vi "Load Calibration Image.vi"(10 "File Path":path=path "C:/ProgramData/Vision/Config/cam6/cam6 calibration.png", 11 "Camera Name":string="Image Calibration 1") -> (0 "error out":errorcluster, 1 "Internal Parameters":T3, 2 "Calibration Axis Info":T2, 3 "Image Out":T1, 4 "Distortion Model Coefficients":T4={"Distortion Model"=-1, "Polynomial Coefficients"={"Radial Coefficients"=[], "Tangential Coefficients"={"P1"=0.0, "P2"=0.0}}, "Division Model kappa"=0.0} {"Distortion Model" items=["None"=-1, "Polynomial"=0, "Division"=1]})   [LabVIEW 2025]
uses:
  <vilib>/vision/Image Controls.llb/IMAQ Image.ctl
  <vilib>/vision/Calibration.llb/Distortion Model Coefficients.ctl
  <vilib>/vision/Calibration.llb/Distortion Model Types.ctl
  <vilib>/vision/Calibration.llb/Internal Parameters.ctl
  <vilib>/vision/NI_Vision_Development_Module.lvlib
panel:
  out "Calibration Camera Image":T1(plugin-control)
  in  "error in":errorcluster
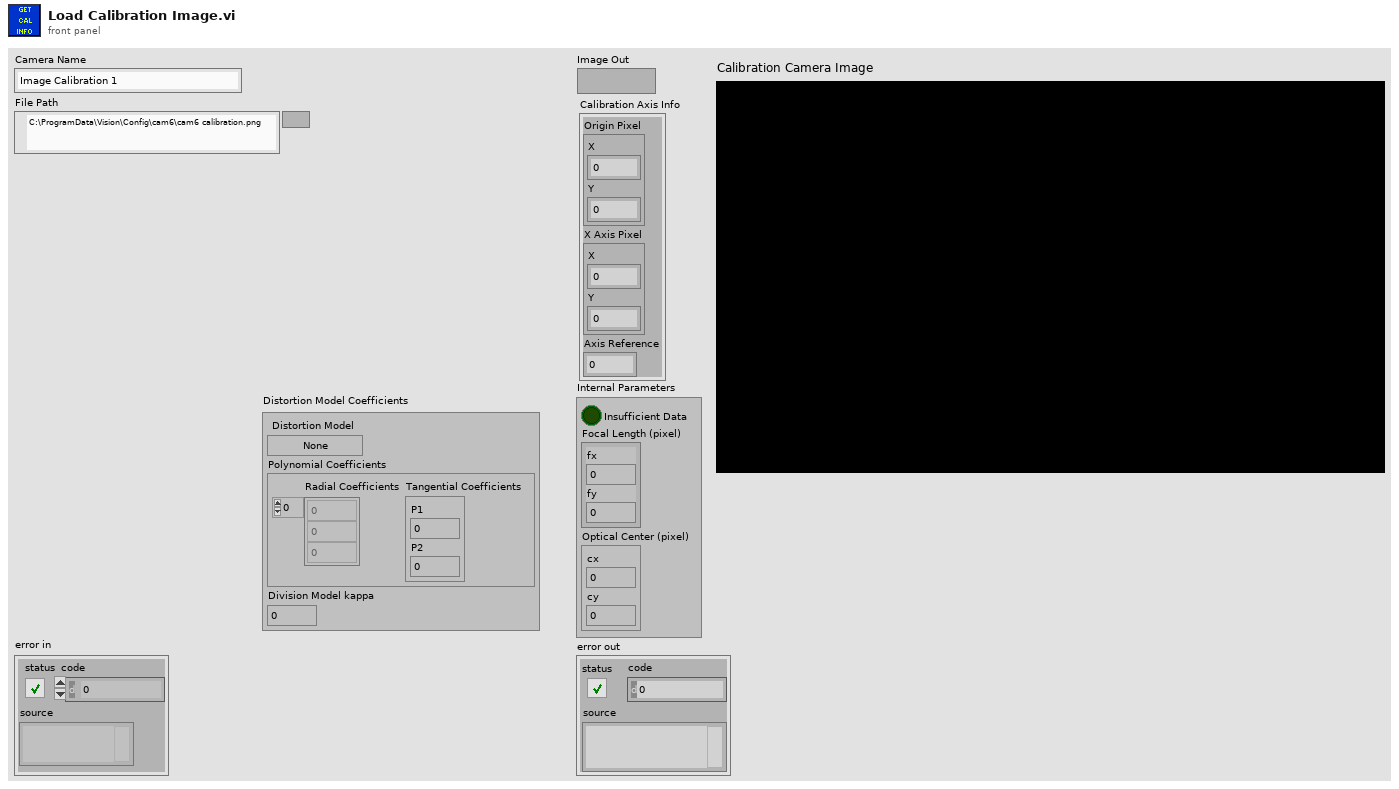
[diagram p1: front panel]
types:
  T1 = typedef "IMAQ Image.ctl" = refnum<image>
  T2 = cluster{"Origin Pixel":cluster{"X":sgl, "Y":sgl}, "X Axis Pixel":cluster{"X":sgl, "Y":sgl}, "Axis Reference":u32}
  T3 = typedef "Internal Parameters.ctl" = cluster{"Insufficient Data":bool, "Focal Length (pixel)":cluster{"fx":sgl, "fy":sgl}, "Optical Center (pixel)":cluster{"cx":sgl, "cy":sgl}}
  T4 = typedef "Distortion Model Coefficients.ctl" = cluster{"Distortion Model":T5, "Polynomial Coefficients":cluster{"Radial Coefficients":sgl[], "Tangential Coefficients":cluster{"P1":sgl, "P2":sgl}}, "Division Model kappa":sgl}
  T5 = typedef "Distortion Model Types.ctl" = i32
  T6 = cluster{"Origin Pixel":cluster{"X":sgl, "Y":sgl}, "Angle Relative to Horizontal (deg)":sgl, "X Axis Pixel":cluster{"X":sgl, "Y":sgl}, "Axis Reference":u32}
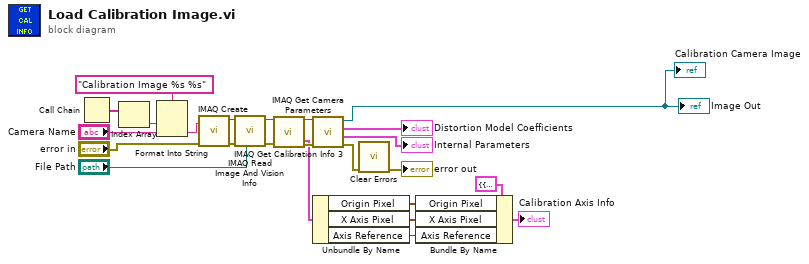
[diagram p0: block diagram]
diagram:
  n1 = Call Chain() -> (call chain=w17:string[])
  n2 = Index Array(array=w17) -> (element=w16:string)  [unwired: 1 in]
  n3 = Format Into String(format string="Calibration Image %s %s" ("Image Name"), w16, "Camera Name") -> ()  [unwired: 2 in, 2 out]
  n4 = call "IMAQ Create"("Image Name"="Camera Name", "error in (no error)"="error in") -> ("New Image"=w19:T1, "error out"=w18:errorcluster)  [unwired: 2 in, 1 out]
  n5 = call "IMAQ Read Image And Vision Info"("File Path"="File Path", "error in (no error)"=w18, "Image"=w19) -> ("error out"=w15:errorcluster, "Image Out"=w13:T1)  [unwired: 1 in, 6 out]
  n6 = call "IMAQ Get Calibration Info 3"("Calibration Template Image"=w13, "error in (no error)"=w15) -> ("Calibration Template Image (duplicate)"=w2:T1, "Calibration Axis Info"=w6:T6, "error out"=w10:errorcluster)  [unwired: 5 in, 6 out]
  n7 = call "IMAQ Get Camera Parameters"("error in (no error)"=w10, "Calibration Template Image"=w2) -> ("error out"=w9:errorcluster, "Internal Parameters"=→"Internal Parameters":T3, "Distortion Model Coefficients"=→"Distortion Model Coefficients":T4, "Calibration Template Image (duplicate)"=→"Image Out" →"Calibration Camera Image":T1)  [unwired: 5 in, 1 out]
  n8 = Unbundle By Name(w6) -> ("Origin Pixel"=w5:cluster{"X":sgl, "Y":sgl}, "X Axis Pixel"=w4:cluster{"X":sgl, "Y":sgl}, "Axis Reference"=w3:u32)
  n9 = call <vilib>:"Clear Errors.vi"("error in (no error)"=w9) -> ("error out"=→"error out":errorcluster)  [unwired: 5 in, 1 out]
  n10 = Bundle By Name(cluster=T2 {"Origin Pixel"={"X"=0.0, "Y"=0.0}, "X Axis Pixel"={"X"=0.0, "Y"=0.0}, "Axis Reference"=1} ("Calibration Axis Info"), "Origin Pixel"=w5, "X Axis Pixel"=w4, "Axis Reference"=w3) -> (→"Calibration Axis Info":T2)
